vi "Car Wash.vi"() -> ()   [LabVIEW 2018]
uses:
  Controls/Car Wash Indicators.ctl
  Controls/Wash Options.ctl
  Controls/States Enum.ctl
  Controls/Timer Mode.ctl
panel:
  in  "Start":bool
  out "Elapsed Time":dbl format="%0.2f"
  in  "Stop":bool
  out "Wash Entry":bool
  in  "Wash Options":T1
  in  "Car Position Slider":u8(slide) max=3 scale=0.0..4.0
  out "Car Wash Indicators":T2
  # "Entry Console"
  # "Car Wash Display"
  # "Car Position Simulation"
  # "Pre-Soak\nH-P Wash\nL-P Wax\nSpot Free Rinse"
  # "Underbody Wash\nBug Remover"
  # "Tire Shine\nAir Dry"
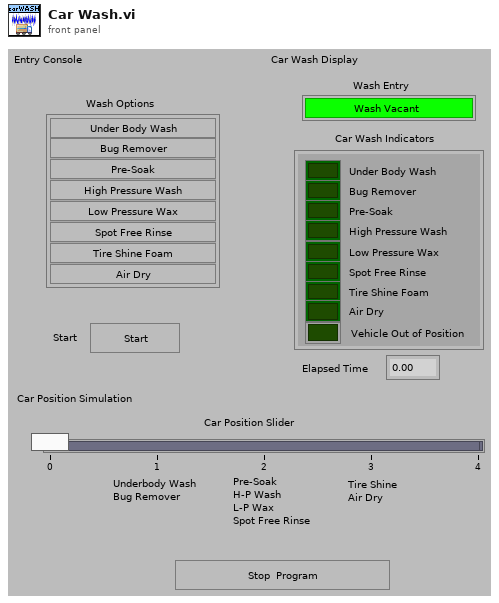
[diagram p1: front panel]
types:
  T1 = typedef "Wash Options.ctl" = cluster{"Underbody Wash":bool, "Bug Remover":bool, "Pre-Soak":bool, "High Pressure Wash":bool, "Low Pressure Wax":bool, "Spot Free Rinse":bool, "Tire Shine Foam":bool, "Air Dry":bool}
  T2 = typedef "Car Wash Indicators.ctl" = cluster{"Under Body Wash":bool, "Bug Remover":bool, "Pre-Soak":bool, "High Pressure Wash":bool, "Low Pressure Wax":bool, "Spot Free Rinse":bool, "Tire Shine Foam":bool, "Air Dry":bool, "Vehicle Out of Position":bool}
  T3 = typedef "States Enum.ctl" = enum16{"Initialize", "WaitEvent", "Stop", "UnderBodyWash", "BugRemover", "PreSoak", "HighPressureWash", "LowPressureWash", "SpotFreeRinse", "TireShineFoam", "AirDry"}
  T4 = enum8{"Enabled", "Disabled", "Disabled and Grayed Out"}
  T5 = enum16{"Entry", "Station 1", "Station 2", "Station 3", "Exit"}
  T6 = typedef "Timer Mode.ctl" = enum16{"Reset", "Get Time", "Start", "Pause"}
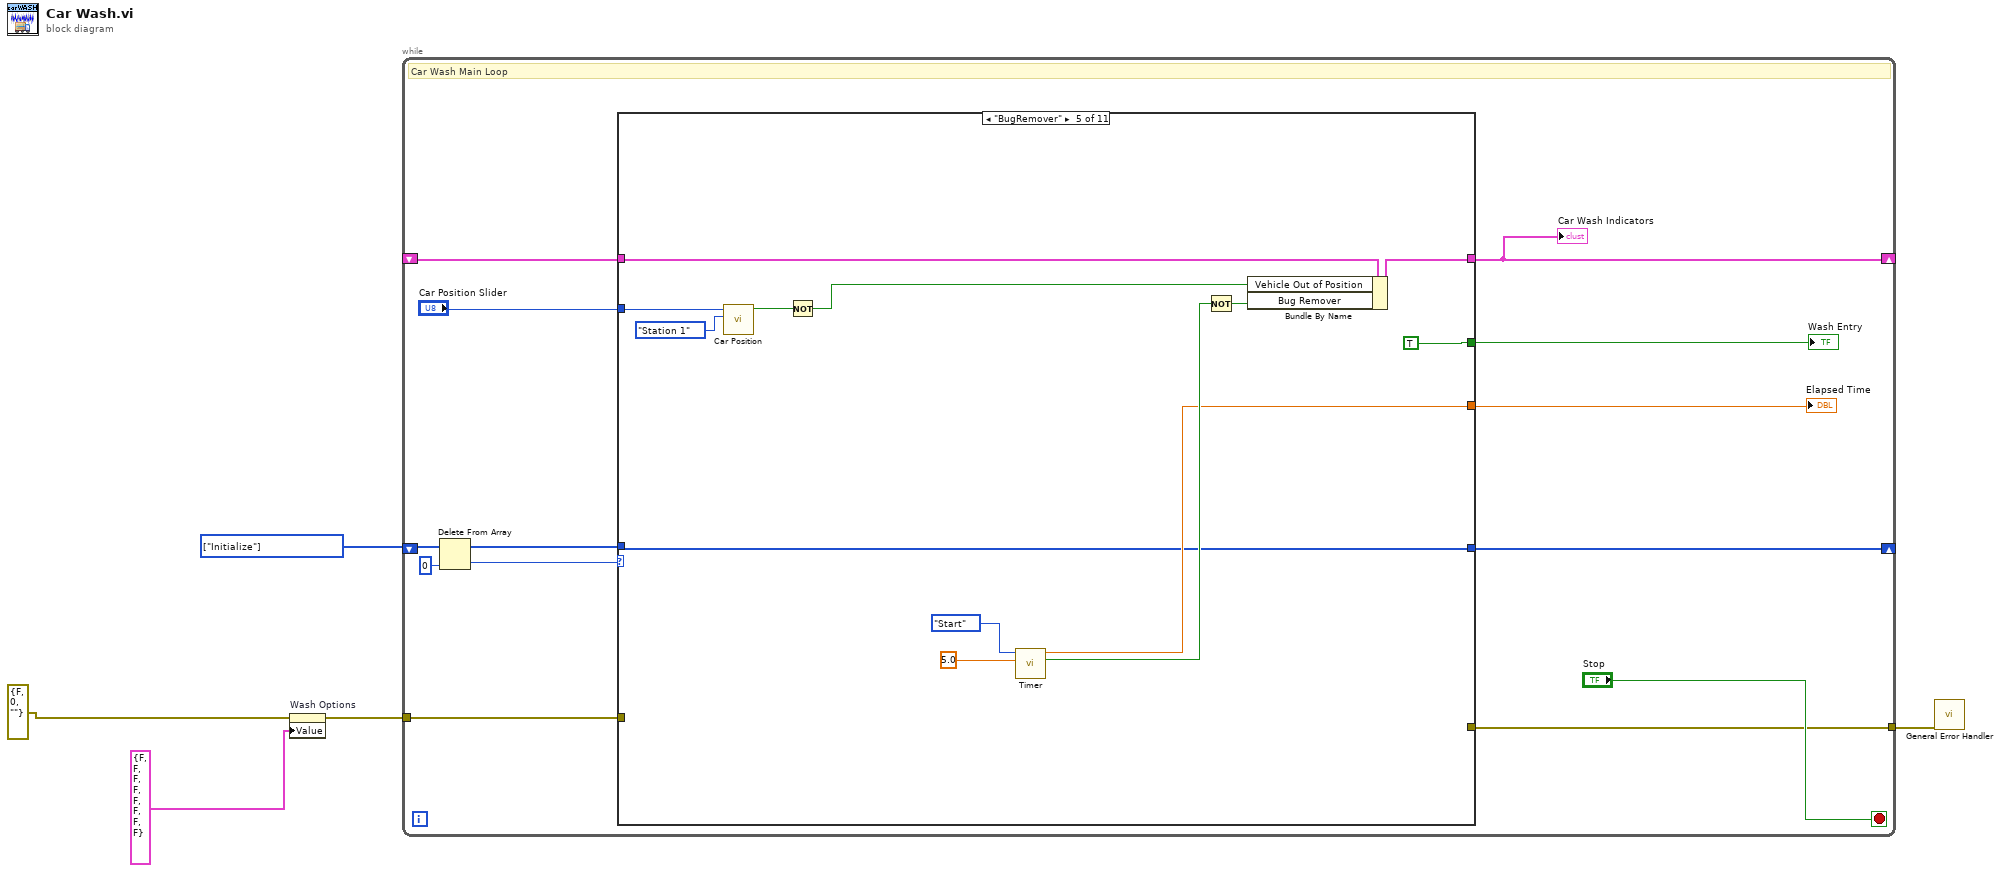
[diagram p0: block diagram]
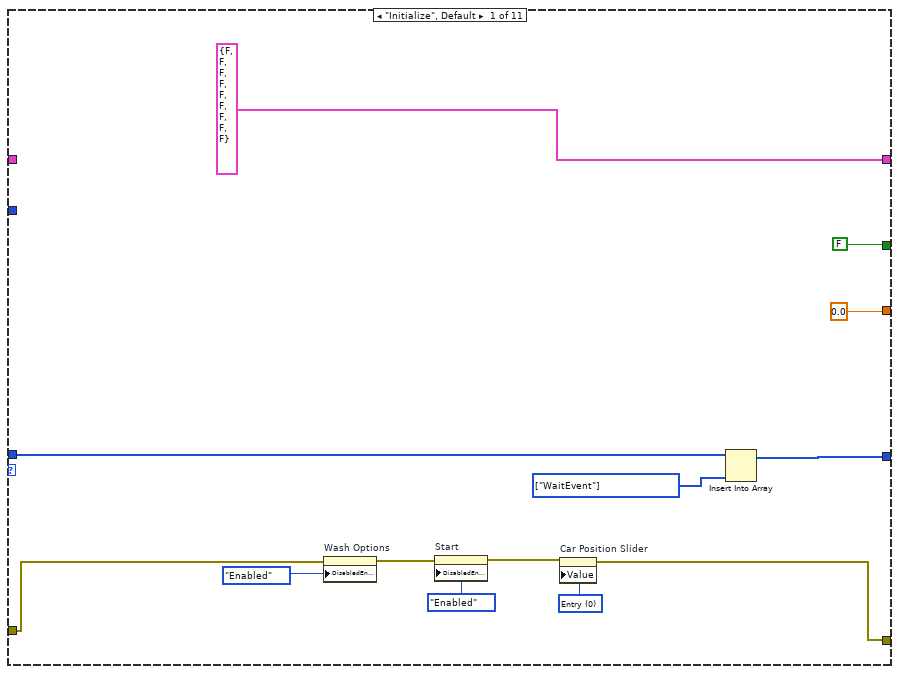
[diagram p2: hidden frame]
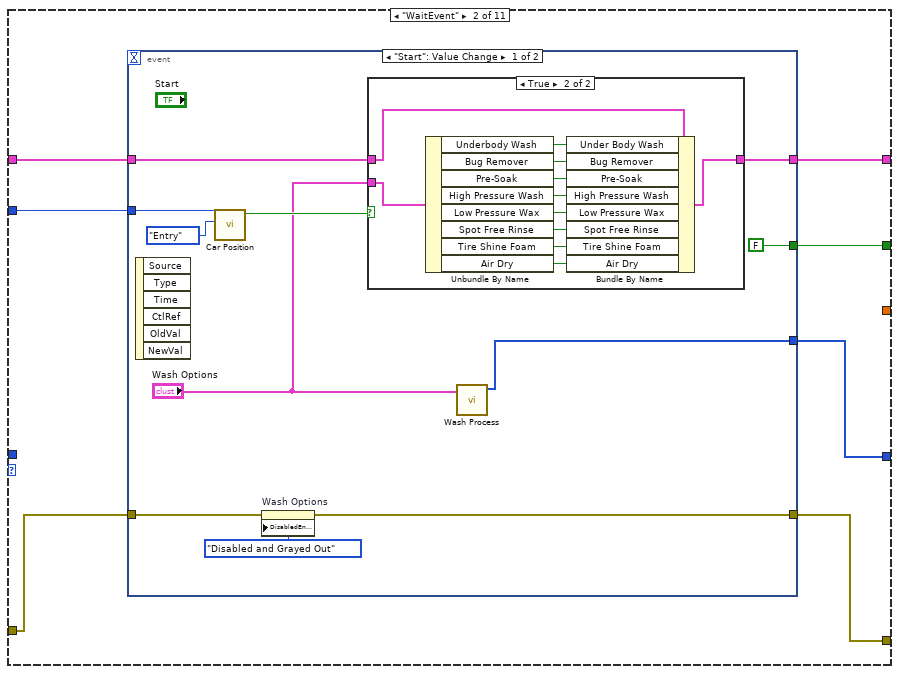
[diagram p3: hidden frame]
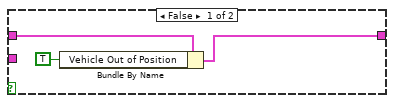
[diagram p4: hidden frame]
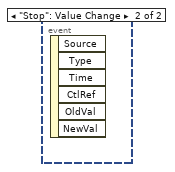
[diagram p5: hidden frame]
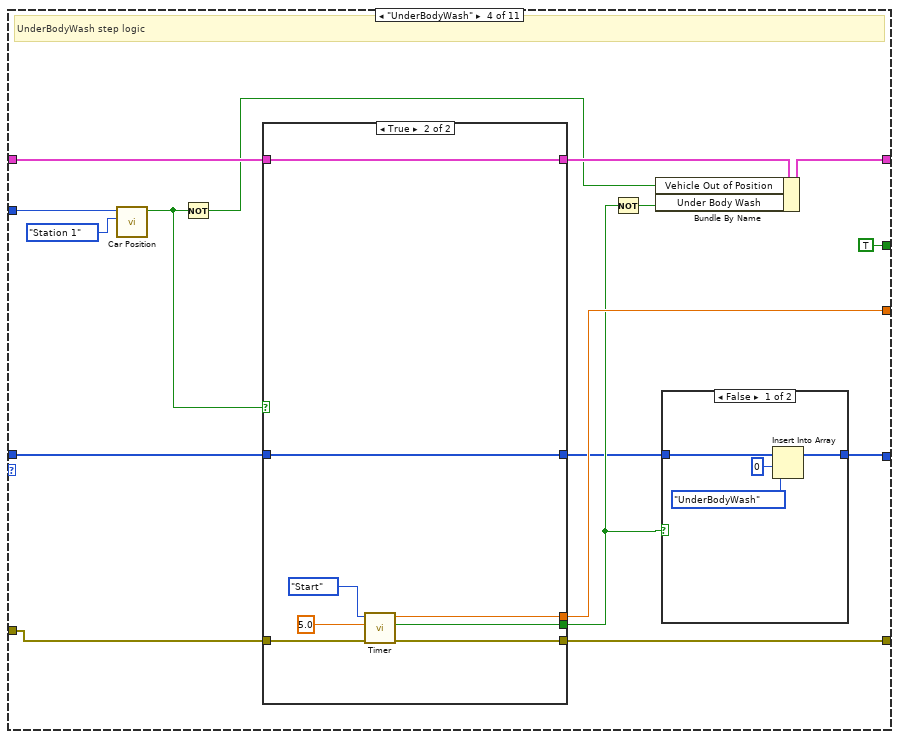
[diagram p7: hidden frame]
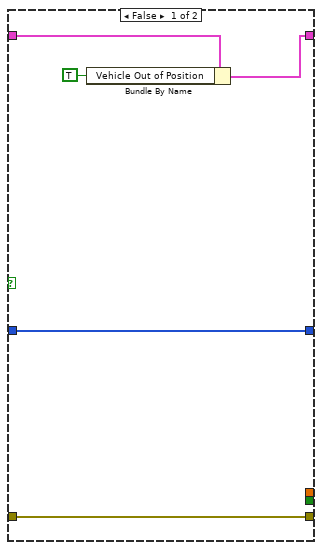
[diagram p9: hidden frame]
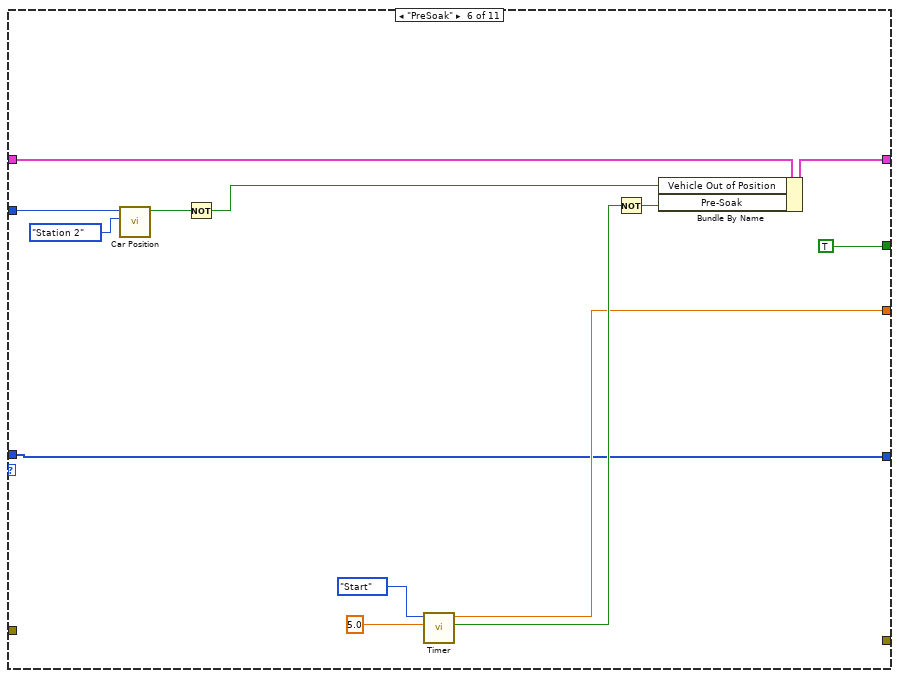
[diagram p10: hidden frame]
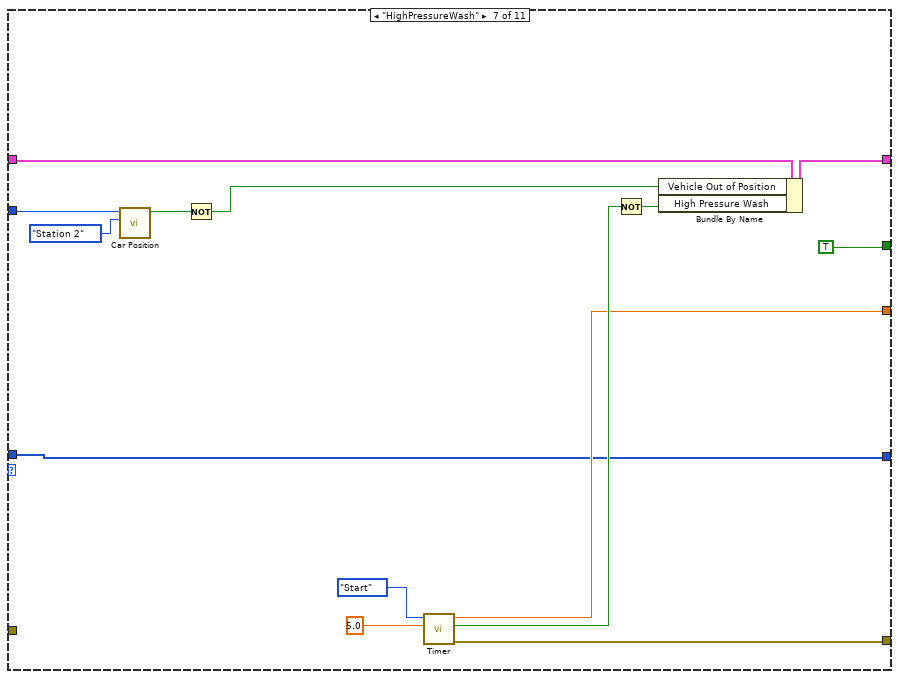
[diagram p11: hidden frame]
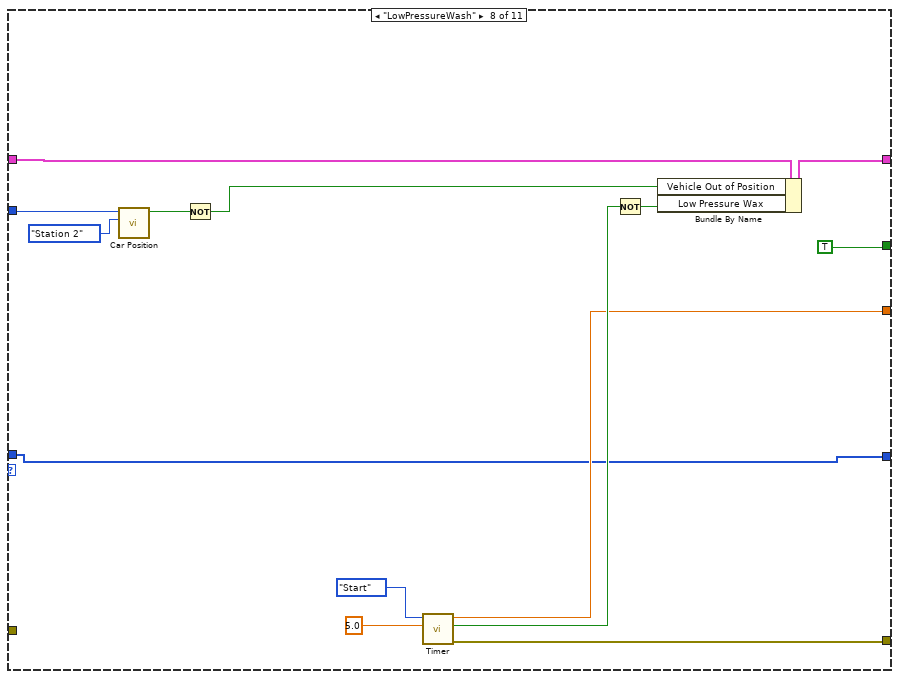
[diagram p12: hidden frame]
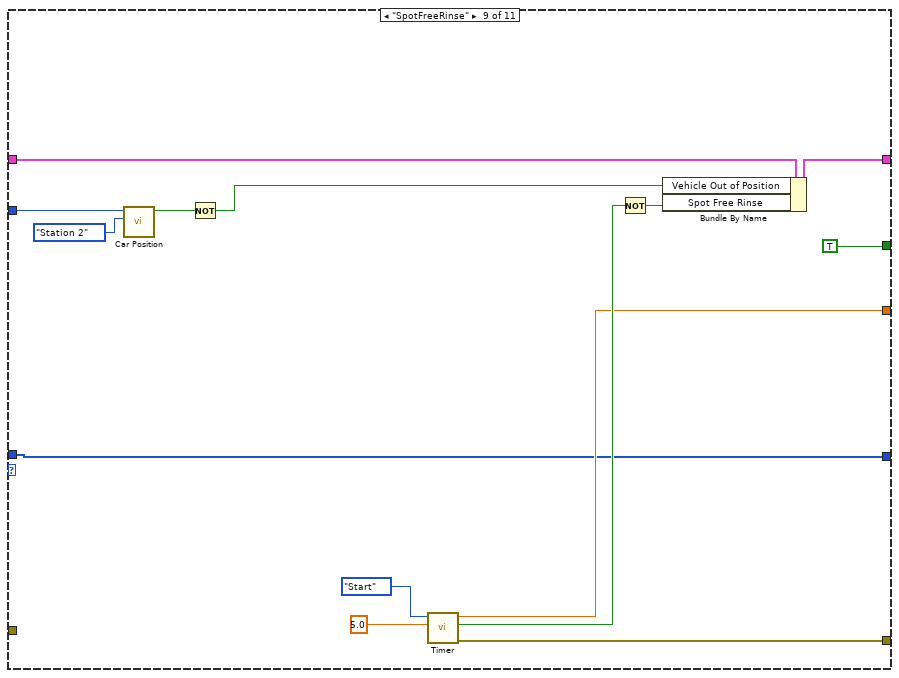
[diagram p13: hidden frame]
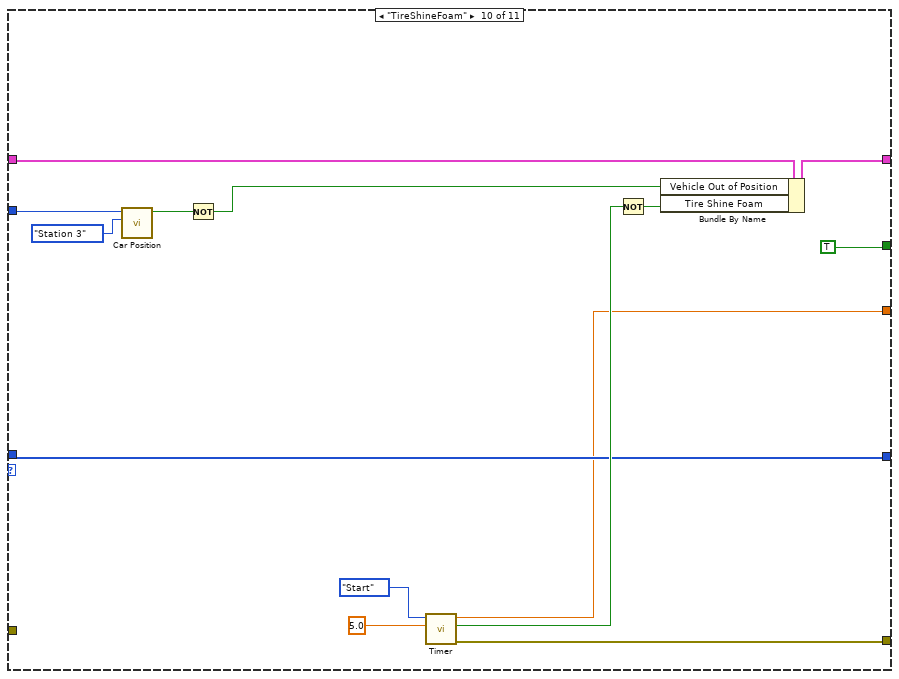
[diagram p14: hidden frame]
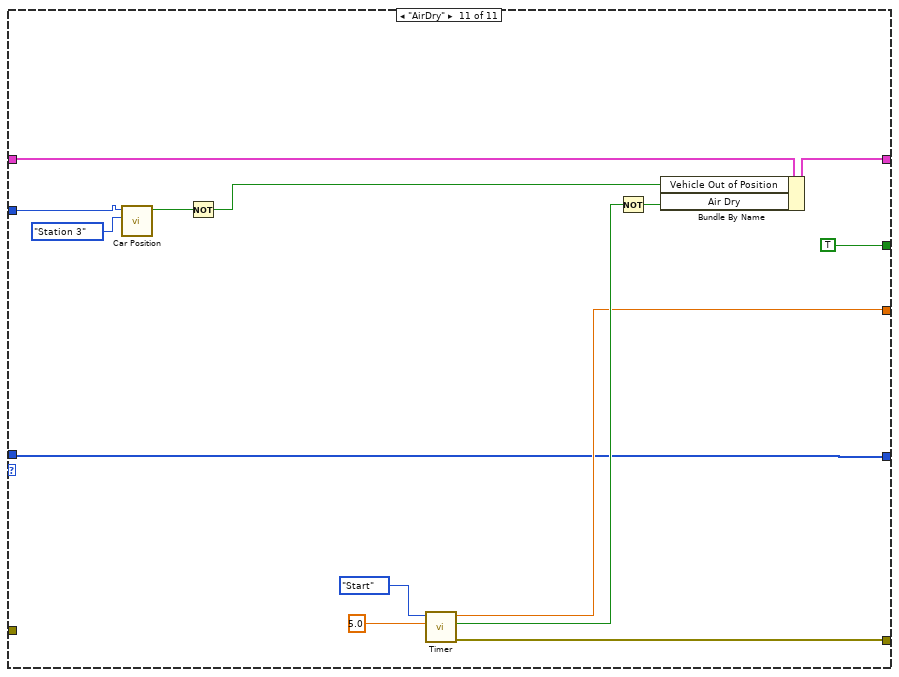
[diagram p15: hidden frame]
diagram:
  w5 = T3[] [enum."Initialize"] items=["Initialize", "WaitEvent", "Stop", "UnderBodyWash", "BugRemover", "PreSoak", "HighPressureWash", "LowPressureWash", "SpotFreeRinse", "TireShineFoam", "AirDry"]
  n1 = property on="Wash Options" class="Clust (strict)"(error in=errorcluster {"status"=FALSE, "code"=0, "source"=""} ("error constant"), "Value"=T1 {"Underbody Wash"=FALSE, "Bug Remover"=FALSE, "Pre-Soak"=FALSE, "High Pressure Wash"=FALSE, "Low Pressure Wax"=FALSE, "Spot Free Rinse"=FALSE, "Tire Shine Foam"=FALSE, "Air Dry"=FALSE} ("Wash Options")) -> (error out=w2:errorcluster)  [unwired: 1 in, 1 out]
  n2 = while {
    shift-right: [w14] -> _
    shift-left: _ -> [w15]
    shift-right: [w9] -> _
    shift-left: w5 -> [w18]
    tunnel: [w7] -> w4
    tunnel: w2 -> [w6]
    stop <- "Stop" stop-if-true
    # "Car Wash Main Loop"
    n3 = Delete From Array(array=w18, index=0) -> (deleted portion=w17:T3, array with subset deleted=w10:T3[])  [unwired: 1 in]
    n4 = case shown="\"BugRemover\"" w17 {
      tunnel: w15 -> [_ w36 _ w73 w103 w117 w131 w145 w159 w173 w187]
      tunnel: [T2 {"Under Body Wash"=FALSE, "Bug Remover"=FALSE, "Pre-Soak"=FALSE, "High Pressure Wash"=FALSE, "Low Pressure Wax"=FALSE, "Spot Free Rinse"=FALSE, "Tire Shine Foam"=FALSE, "Air Dry"=FALSE, "Vehicle Out of Position"=FALSE} ("Car Wash Indicators") w34 _ w78 w102 w115 w129 w143 w158 w172 w184] -> w14
      tunnel: [FALSE w37 _ TRUE TRUE TRUE TRUE TRUE TRUE TRUE TRUE] -> w13
      tunnel: [0.0 _ _ w76 w101 w113 w127 w141 w156 w168 w183] -> w12
      tunnel: w10 -> [w23 _ w64 w71 w100 w112 w126 w140 w155 w170 w182]
      tunnel: [w21 w38 w64 w67 w100 w112 w126 w140 w155 w170 w182] -> w9
      tunnel: "Car Position Slider" -> [_ w35 _ w80 w104 w116 w130 w144 w153 w167 w186]
      tunnel: [w20 w32 _ w77 _ _ w125 w139 w154 w169 w181] -> w7
      tunnel: w6 -> [w19 w33 _ w70 _ _ _ _ _ _ _]
      frame "Initialize", Default {
        w22 = T3[] [enum."WaitEvent"] items=["Initialize", "WaitEvent", "Stop", "UnderBodyWash", "BugRemover", "PreSoak", "HighPressureWash", "LowPressureWash", "SpotFreeRinse", "TireShineFoam", "AirDry"]
        w25 = u8 0 items=["Entry", "Station 1", "Station 2", "Station 3", "Exit"] ("Car Position Slider")
        n5 = property on="Wash Options" class="Clust (strict)"(error in=w19, "DisabledEnum"=T4."Enabled" ("Disabled")) -> (error out=w28:errorcluster)  [unwired: 1 in, 1 out]
        n6 = property on="Start" class="Bool"(error in=w28, "DisabledEnum"=T4."Enabled" ("Disabled")) -> (error out=w24:errorcluster)  [unwired: 1 in, 1 out]
        n7 = property on="Car Position Slider" class="Slide (strict)"(error in=w24, "Value"=w25) -> (error out=w20:errorcluster)  [unwired: 1 in, 1 out]
        n8 = Insert Into Array(array=w23, new element=w22) -> (w21:T3[])  [unwired: 1 in]
      }
      frame "WaitEvent" {
        n9 = event shown="[0] \"Start\": Value Change" {
          selector: _ -> [_ _]
          dyn-events: _ -> [_ _]
          timeout: _ -> [_ _]
          tunnel: [w41 _] -> w38
          tunnel: [FALSE _] -> w37
          tunnel: w36 -> [w45 _]
          tunnel: w35 -> [w47 _]
          tunnel: [w44 _] -> w34
          tunnel: w33 -> [w40 _]
          tunnel: [w39 _] -> w32
          event "Start": Value Change {
            n10 = event-data() -> ()  [unwired: 1 in, 6 out]
            n11 = call "Car Position.vi"("Position Needed"=T5."Entry", "Car Position Slider"=w47) -> ("In Position"=w43:bool)  [unwired: 9 in]
            n12 = property on="Wash Options" class="Clust (strict)"(error in=w40, "DisabledEnum"=T4."Disabled and Grayed Out" ("Disabled")) -> (error out=w39:errorcluster)  [unwired: 1 in, 1 out]
            n13 = case shown="True" w43 {
              tunnel: w45 -> [w52 w62]
              tunnel: [w51 w61] -> w44
              tunnel: "Wash Options" -> [_ w63]
              frame False {
                n14 = Bundle By Name(cluster=w52, "Vehicle Out of Position"=TRUE) -> (w51:T2)
              }
              frame True {
                n15 = Unbundle By Name(w63) -> ("Underbody Wash"=w60:bool, "Bug Remover"=w59:bool, "Pre-Soak"=w58:bool, "High Pressure Wash"=w57:bool, "Low Pressure Wax"=w56:bool, "Spot Free Rinse"=w55:bool, "Tire Shine Foam"=w54:bool, "Air Dry"=w53:bool)
                n16 = Bundle By Name(cluster=w62, "Under Body Wash"=w60, "Bug Remover"=w59, "Pre-Soak"=w58, "High Pressure Wash"=w57, "Low Pressure Wax"=w56, "Spot Free Rinse"=w55, "Tire Shine Foam"=w54, "Air Dry"=w53) -> (w61:T2)
              }
            }
            n17 = call "Wash Process.vi"("Wash Options"="Wash Options") -> ("Array"=w41:T3[])  [unwired: 10 in]
          }
          event "Stop": Value Change {
            n18 = event-data() -> ()  [unwired: 1 in, 6 out]
          }
        }
      }
      frame "Stop" {
      }
      frame "UnderBodyWash" {
        # "UnderBodyWash step logic"
        n19 = call "Car Position.vi"("Position Needed"=T5."Station 1", "Car Position Slider"=w80) -> ("In Position"=w65:bool)  [unwired: 9 in]
        n20 = Not(x=w65) -> (.not. x?=w66:bool)
        n21 = case shown="True" w65 {
          tunnel: [w86 w96] -> w77
          tunnel: [_ w95] -> w76
          tunnel: [_ w94] -> w69
          tunnel: w73 -> [w89 w93]
          tunnel: [w88 w93] -> w72
          tunnel: w71 -> [w90 w92]
          tunnel: [w90 w92] -> w68
          tunnel: w70 -> [w86 w91]
          frame False {
            n22 = Bundle By Name(cluster=w89, "Vehicle Out of Position"=TRUE) -> (w88:T2)
          }
          frame True {
            n23 = call "Timer.vi"("error in"=w91, "Time Target"=5.0, "Timer Mode"=Timer_Mode."Start") -> ("error out"=w96:errorcluster, "Time Has Elapsed"=w94:bool, "Elapsed Time (s)"=w95:dbl)  [unwired: 6 in]
          }
        }
        n24 = Not(x=w69) -> (.not. x?=w74:bool)
        n25 = Bundle By Name(cluster=w72, "Vehicle Out of Position"=w66, "Under Body Wash"=w74) -> (w78:T2)
        n26 = case shown="False" w69 {
          tunnel: w68 -> [w84 w85]
          tunnel: [w81 w85] -> w67
          frame False {
            n27 = Insert Into Array(array=w84, index=0, new element=States_Enum."UnderBodyWash" ("new element/subarray")) -> (w81:T3[])
          }
          frame True {
          }
        }
      }
      frame "BugRemover" {
        n28 = call "Car Position.vi"("Position Needed"=T5."Station 1", "Car Position Slider"=w104) -> ("In Position"=w109:bool)  [unwired: 9 in]
        n29 = Not(x=w109) -> (.not. x?=w110:bool)
        n30 = call "Timer.vi"("Time Target"=5.0, "Timer Mode"=Timer_Mode."Start") -> ("Time Has Elapsed"=w105:bool, "Elapsed Time (s)"=w101:dbl)  [unwired: 7 in, 1 out]
        n31 = Not(x=w105) -> (.not. x?=w106:bool)
        n32 = Bundle By Name(cluster=w103, "Vehicle Out of Position"=w110, "Bug Remover"=w106) -> (w102:T2)
      }
      frame "PreSoak" {
        n33 = call "Car Position.vi"("Position Needed"=T5."Station 2", "Car Position Slider"=w116) -> ("In Position"=w122:bool)  [unwired: 9 in]
        n34 = Not(x=w122) -> (.not. x?=w123:bool)
        n35 = call "Timer.vi"("Time Target"=5.0, "Timer Mode"=Timer_Mode."Start") -> ("Time Has Elapsed"=w118:bool, "Elapsed Time (s)"=w113:dbl)  [unwired: 7 in, 1 out]
        n36 = Not(x=w118) -> (.not. x?=w119:bool)
        n37 = Bundle By Name(cluster=w117, "Vehicle Out of Position"=w123, "Pre-Soak"=w119) -> (w115:T2)
      }
      frame "HighPressureWash" {
        n38 = call "Car Position.vi"("Position Needed"=T5."Station 2", "Car Position Slider"=w130) -> ("In Position"=w136:bool)  [unwired: 9 in]
        n39 = Not(x=w136) -> (.not. x?=w137:bool)
        n40 = call "Timer.vi"("Time Target"=5.0, "Timer Mode"=Timer_Mode."Start") -> ("error out"=w125:errorcluster, "Time Has Elapsed"=w132:bool, "Elapsed Time (s)"=w127:dbl)  [unwired: 7 in]
        n41 = Not(x=w132) -> (.not. x?=w133:bool)
        n42 = Bundle By Name(cluster=w131, "Vehicle Out of Position"=w137, "High Pressure Wash"=w133) -> (w129:T2)
      }
      frame "LowPressureWash" {
        n43 = call "Car Position.vi"("Position Needed"=T5."Station 2", "Car Position Slider"=w144) -> ("In Position"=w150:bool)  [unwired: 9 in]
        n44 = Not(x=w150) -> (.not. x?=w151:bool)
        n45 = call "Timer.vi"("Time Target"=5.0, "Timer Mode"=Timer_Mode."Start") -> ("error out"=w139:errorcluster, "Time Has Elapsed"=w146:bool, "Elapsed Time (s)"=w141:dbl)  [unwired: 7 in]
        n46 = Not(x=w146) -> (.not. x?=w147:bool)
        n47 = Bundle By Name(cluster=w145, "Vehicle Out of Position"=w151, "Low Pressure Wax"=w147) -> (w143:T2)
      }
      frame "SpotFreeRinse" {
        n48 = call "Car Position.vi"("Position Needed"=T5."Station 2", "Car Position Slider"=w153) -> ("In Position"=w164:bool)  [unwired: 9 in]
        n49 = Not(x=w164) -> (.not. x?=w165:bool)
        n50 = call "Timer.vi"("Time Target"=5.0, "Timer Mode"=Timer_Mode."Start") -> ("error out"=w154:errorcluster, "Time Has Elapsed"=w160:bool, "Elapsed Time (s)"=w156:dbl)  [unwired: 7 in]
        n51 = Not(x=w160) -> (.not. x?=w161:bool)
        n52 = Bundle By Name(cluster=w159, "Vehicle Out of Position"=w165, "Spot Free Rinse"=w161) -> (w158:T2)
      }
      frame "TireShineFoam" {
        n53 = call "Car Position.vi"("Position Needed"=T5."Station 3", "Car Position Slider"=w167) -> ("In Position"=w178:bool)  [unwired: 9 in]
        n54 = Not(x=w178) -> (.not. x?=w179:bool)
        n55 = call "Timer.vi"("Time Target"=5.0, "Timer Mode"=Timer_Mode."Start") -> ("error out"=w169:errorcluster, "Time Has Elapsed"=w174:bool, "Elapsed Time (s)"=w168:dbl)  [unwired: 7 in]
        n56 = Not(x=w174) -> (.not. x?=w175:bool)
        n57 = Bundle By Name(cluster=w173, "Vehicle Out of Position"=w179, "Tire Shine Foam"=w175) -> (w172:T2)
      }
      frame "AirDry" {
        n58 = call "Car Position.vi"("Position Needed"=T5."Station 3", "Car Position Slider"=w186) -> ("In Position"=w192:bool)  [unwired: 9 in]
        n59 = Not(x=w192) -> (.not. x?=w193:bool)
        n60 = call "Timer.vi"("Time Target"=5.0, "Timer Mode"=Timer_Mode."Start") -> ("error out"=w181:errorcluster, "Time Has Elapsed"=w188:bool, "Elapsed Time (s)"=w183:dbl)  [unwired: 7 in]
        n61 = Not(x=w188) -> (.not. x?=w189:bool)
        n62 = Bundle By Name(cluster=w187, "Vehicle Out of Position"=w193, "Air Dry"=w189) -> (w184:T2)
      }
    }
    "Car Wash Indicators" <- w14
    "Wash Entry" <- w13
    "Elapsed Time" <- w12
  }
  n63 = call <vilib>:"General Error Handler.vi"("error in (no error)"=w4) -> ()  [unwired: 10 in, 5 out]
